vi "CN Dislay.vi"(8 "error in (no error)":errorcluster, 10 "CN image":T1, 11 "output array":refnum<vi>[](array[refnum])) -> (0 "error out":errorcluster)   [LabVIEW 2014]
uses:
  Type'def/CN image Ctr.ctl
  <vilib>/picture/picture.llb/imagedata.ctl
  Type'def/CN Config Ctr.ctl
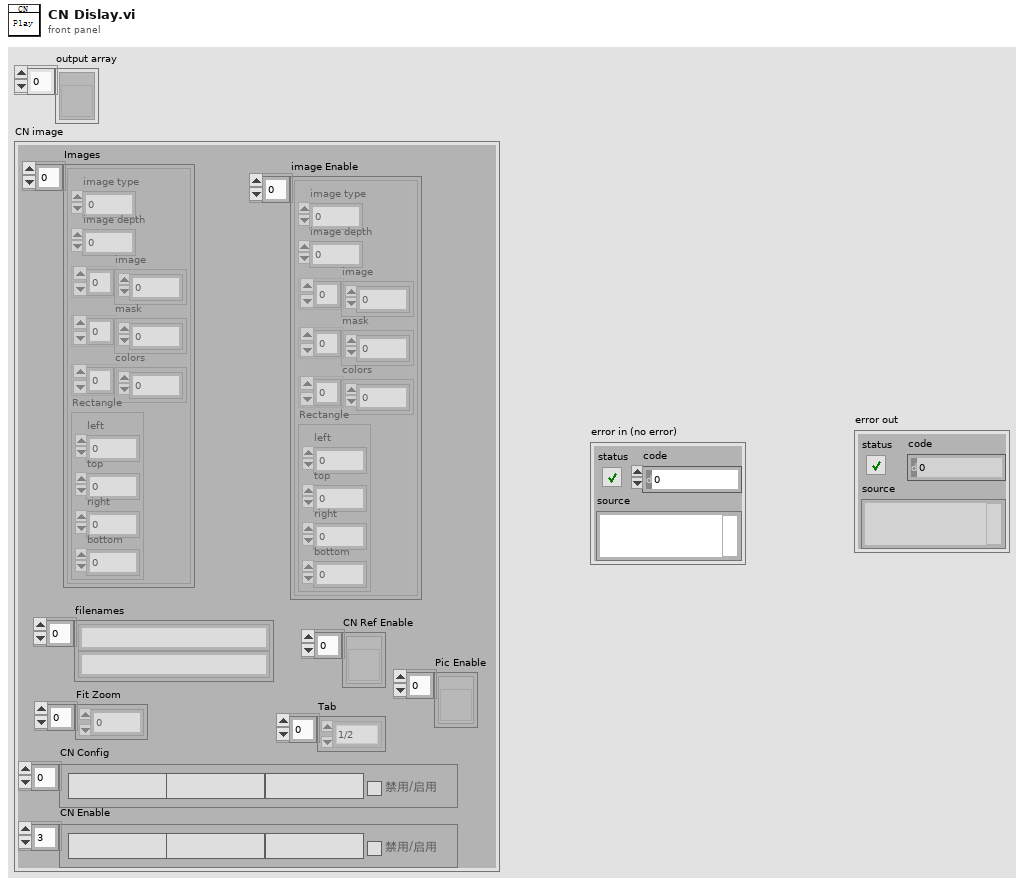
[diagram p1: front panel]
types:
  T1 = typedef "CN image Ctr.ctl" = cluster{"Images":T2[], "filenames":string[], "Fit Zoom":dbl[], "CN Config":T3[], "CN Enable":T3[], "image Enable":T2[], "CN Ref Enable":refnum<vi>[], "Tab ":enum32{"1/2", "1/3", "1/4", "1/5", "2/5", "3/5"}[], "Pic Enable":refnum<vi>[]}
  T2 = typedef "imagedata.ctl" = cluster{"image type":i32, "image depth":i32, "image":u8[], "mask":u8[], "colors":u32[], "Rectangle":cluster{"left":i16, "top":i16, "right":i16, "bottom":i16}}
  T3 = typedef "CN Config Ctr.ctl" = cluster{"Model":string, "Pic_Name":string, "CarName":string, "En/Disable":bool}
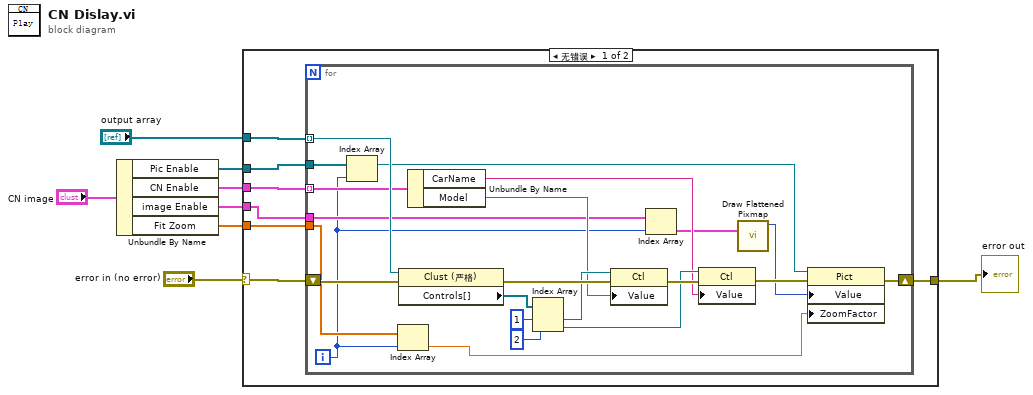
[diagram p0: block diagram]
diagram:
  n1 = Unbundle By Name("CN image") -> ("Pic Enable"=w4:refnum<vi>[], "CN Enable"=w5:T3[], "image Enable"=w3:T2[], "Fit Zoom"=w2:dbl[])
  n2 = case shown="无错误" "error in (no error)" {
    selector: "error in (no error)" -> [w14 w38]
    tunnel: "output array" -> [w15 _]
    tunnel: w5 -> [w13 _]
    tunnel: w4 -> [w12 _]
    tunnel: w3 -> [w11 _]
    tunnel: w2 -> [w10 _]
    tunnel: [w9 w38] -> w1
    frame No Error {
      n3 = for {
        tunnel: w15 -> [w36] mode=indexing
        tunnel: w13 -> [w30] mode=indexing
        tunnel: w12 -> [w24]
        tunnel: w11 -> [w20]
        tunnel: w10 -> [w19]
        shift-right: [w16] -> w9
        shift-left: w14 -> [w37]
        i -> [w18]
        n4 = Index Array(array=w24, index=w18) -> (element=w23:refnum<vi>)
        n5 = Index Array(array=w19, index=w18) -> (element=w17:dbl)
        n6 = property class="Clust (严格)"(reference=w36, error in=w37) -> (error out=w32:errorcluster, "Controls[]"=w35:refnum<vi>[])  [unwired: 1 out]
        n7 = Unbundle By Name(w30) -> ("CarName"=w26:string, "Model"=w29:string)
        n8 = Index Array(array=w35, index #1=1 ("index"), index #2=2 ("index")) -> (element #1=w31:refnum<vi>, element #2=w27:refnum<vi>)
        n9 = property class="Ctl"(reference=w31, error in=w32, "Value"=w29) -> (error out=w28:errorcluster)  [unwired: 1 out]
        n10 = Index Array(array=w20, index=w18) -> (element=w21:T2)
        n11 = property class="Ctl"(reference=w27, error in=w28, "Value"=w26) -> (error out=w25:errorcluster)  [unwired: 1 out]
        n12 = call <vilib>:"Draw Flattened Pixmap.vi"("image data"=w21) -> ("new picture"=w22:picture)  [unwired: 8 in]
        n13 = property class="Pict"(reference=w23, error in=w25, "Value"=w22, "ZoomFactor"=w17) -> (error out=w16:errorcluster)  [unwired: 1 out]
      }
    }
    frame Error {
    }
  }
  "error out" <- w1
